vi "Get Package Details.vi"(7 "LabVIEW Web Service Request":refnum<class "Web Request.lvclass">) -> ()   [LabVIEW 2016]
uses:
  <vilib>/wsapi/Web Request.lvclass
  Packages/Repo_class/Repo.lvclass/Repo.ctl
  Packages/Package_class/Package.lvclass/Package.ctl
  Packages/Package Version_class/Package Version.lvclass/Package Version.ctl
  Packages/Package Version_class/Read Version Text.vi
  Packages/Package_class/Read Versions.vi
  Packages/Package_class/Read Name.vi
  Packages/Repo_class/Read Packages.vi
  GV_Repos.vi
  Packages/Package_class/Package.lvclass
  Packages/Package Version_class/Package Version.lvclass
  WSsupport.lvlib
  Packages/Repo_class/Repo.lvclass
  ServerErrors/ServerErrors.lvlib
panel:
  # "Use the Web Service Request input terminal to call the VIs on the Web Services palette. Do not remove it from the connector pane unless you don't need access to the palette."
  # "Each additional control wired to the connector pane will be available as an input in the URL. To include an indicator in terminal-mode output (the default setting), it must also be wired to the connector pane."
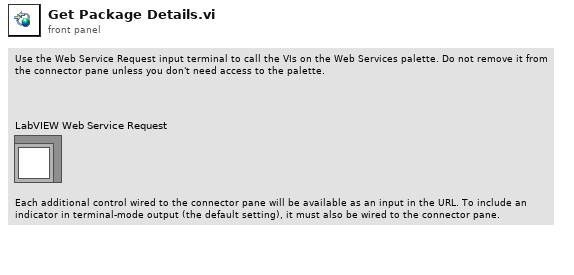
[diagram p1: front panel]
types:
  T1 = typedef "ServerErrors.lvlib/Error Message--cluster.ctl" = cluster{"HTTP Code":i32, "JSON Response":cluster{"error":string, "reason":string}}
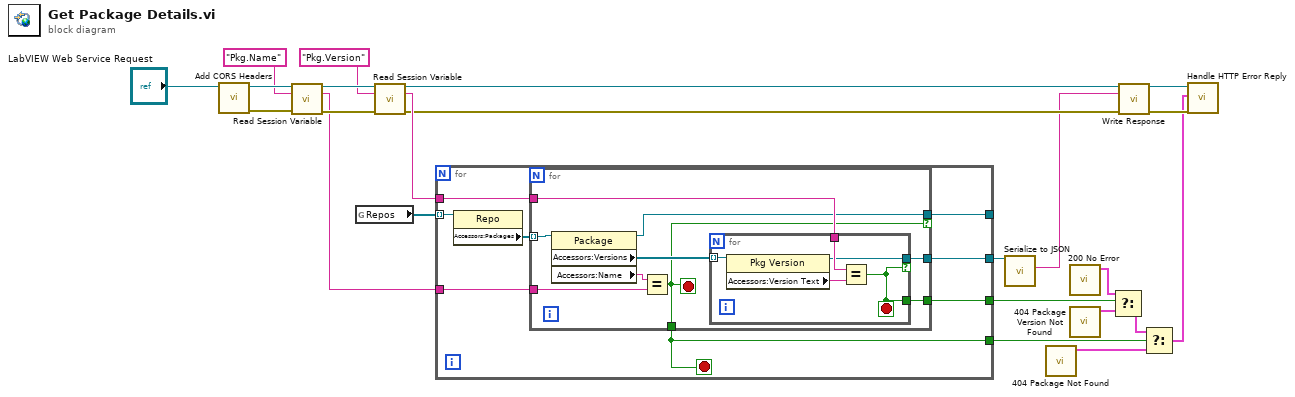
[diagram p0: block diagram]
diagram:
  n1 = call "Add CORS Headers.vi"("LabVIEW Web Service Request"="LabVIEW Web Service Request") -> ("error out"=w21:errorcluster, "LabVIEW Web Service Request out"=w22:refnum<class "Web Request.lvclass">)  [unwired: 9 in]
  n2 = call <vilib>:"Read Session Variable.vi"("LabVIEW Web Service Request"=w22, "key"="Pkg.Name", "error in (no error)"=w21) -> ("LabVIEW Web Service Request out"=w19:refnum<class "Web Request.lvclass">, "value"=w15:string, "error out"=w18:errorcluster)  [unwired: 10 in]
  n3 = global read "GV_Repos.vi" "Repos"() -> (w16:refnum<class "Repo.lvclass">[])
  n4 = call <vilib>:"Read Session Variable.vi"("LabVIEW Web Service Request"=w19, "key"="Pkg.Version", "error in (no error)"=w18) -> ("LabVIEW Web Service Request out"=w12:refnum<class "Web Request.lvclass">, "value"=w14:string, "error out"=w11:errorcluster)  [unwired: 10 in]
  n5 = for {
    tunnel: w16 -> [w31] mode=indexing
    tunnel: w15 -> [w29]
    tunnel: w14 -> [w28]
    tunnel: [w27] -> w13
    tunnel: [w26] -> _
    tunnel: [w24] -> w7
    tunnel: [w25] -> w5
    stop <- w24 stop-if-true
    n6 = property class="Repo"(reference=w31) -> ("Accessors:Packages"=w30:refnum<class "Package.lvclass">[])  [unwired: 1 in, 2 out]
    n7 = for {
      tunnel: w30 -> [w40] mode=indexing
      tunnel: w29 -> [w38]
      tunnel: [w33] -> w24
      tunnel: w28 -> [w36]
      tunnel: [w35] -> w27
      tunnel: [w34] -> w26 if=w33
      tunnel: [w32] -> w25
      stop <- w33 stop-if-true
      n8 = property class="Package"(reference=w40) -> (reference out=w34:refnum<class "Package.lvclass">, "Accessors:Versions"=w37:refnum<class "Package Version.lvclass">[], "Accessors:Name"=w39:string)  [unwired: 1 in, 1 out]
      n9 = Equal?(x=w39, y=w38) -> (x = y?=w33:bool)
      n10 = for {
        tunnel: w37 -> [w45] mode=indexing
        tunnel: w36 -> [w43]
        tunnel: [w42] -> w35 if=w41
        tunnel: [w41] -> w32
        stop <- w41 stop-if-true
        n11 = property class="Pkg Version"(reference=w45) -> (reference out=w42:refnum<class "Package Version.lvclass">, "Accessors:Version Text"=w44:string)  [unwired: 1 in, 1 out]
        n12 = Equal?(x=w43, y=w44) -> (x = y?=w41:bool)
      }
    }
  }
  n13 = call-dynamic "Serialize to JSON.vi"("Pkg Details in"=w13) -> ("JSON string"=w10:string)  [unwired: 7 in, 3 out]
  n14 = call "404 Package Not Found.vi"() -> ("error"=w6:T1)  [unwired: 11 in]
  n15 = call "200 No Error.vi"() -> ("no error"=w4:T1)  [unwired: 11 in]
  n16 = call "404 Package Version Not Found.vi"() -> ("error"=w3:T1)  [unwired: 11 in]
  n17 = Select(t=w4, s=w5, f=w3) -> (s? t:f=w2:T1)
  n18 = call <vilib>:"Write Response.vi"("LabVIEW Web Service Request"=w12, "response string"=w10, "error in (no error)"=w11) -> ("LabVIEW Web Service Request out"=w9:refnum<class "Web Request.lvclass">, "error out"=w8:errorcluster)  [unwired: 11 in]
  n19 = Select(t=w2, s=w7, f=w6) -> (s? t:f=w1:T1)
  n20 = call "Handle HTTP Error Reply.vi"("error in (no error)"=w8, "HTTP Status Code"=w1, "Web Request in"=w9) -> ()  [unwired: 8 in, 1 out]
